vi "Choreo_Trajectory_SampleInternal.vi"(9 "TimeStamp":dbl, 11 "ChoreoTrajectory":T2) -> (3 "ChoreoTrajectoryState":T1)   [LabVIEW 2019, in "ChoreoLib.lvlib"]
doc: "This is an internal routine. It should NOT be called by the end user. Return an interpolated sample of the trajectory at the given timestamp.\n\nInputs: \n - ChoreoTrajectory - cluster - The trajectory to sample.\n - timestamp - double - The timestamp of this sample relative to the beginning of the trajectory.\n\nOutputs:\n - ChoreoTrajectoryState - cluster - The ChoreoTrajectoryState at the given time."
uses:
  ChoreoLib.lvlib
  TypeDef/ChoreoTrajectory.ctl
  TypeDef/ChoreoTrajectoryState.ctl
  Choreo_TrajectoryState_New.vi
  Choreo_TrajectoryState_GetAll.vi
  <vilib>/Rock Robotics/WPI/ThirdParty/JAS_Junk/TrajLib/Pose2d_Interpolate.vi
  Choreo_TrajectoryState_GetPose.vi
  <vilib>/Rock Robotics/WPI/ThirdParty/JAS_Junk/TrajLib/MathUtil_Interpolate.vi
  <vilib>/Rock Robotics/WPI/ThirdParty/JAS_Junk/TrajLib/Pose2d_getXYAngle.vi
  <vilib>/Rock Robotics/WPI/ThirdParty/JAS_Junk/TrajLib/Twist2d_GetAll.vi
  <vilib>/Rock Robotics/WPI/ThirdParty/JAS_Junk/TrajLib/Twist2d_Create.vi
  <vilib>/Rock Robotics/WPI/ThirdParty/JAS_Junk/TrajLib/Pose2d_New.vi
  <vilib>/Rock Robotics/WPI/ThirdParty/JAS_Junk/TrajLib/MathUtil_Clamp.vi
  <vilib>/Rock Robotics/WPI/ThirdParty/JAS_Junk/TrajLib/Rotation2d_CreateAngle.vi
  <vilib>/Rock Robotics/WPI/ThirdParty/JAS_Junk/TrajLib/Translation2d_Create.vi
  <vilib>/Rock Robotics/WPI/ThirdParty/JAS_Junk/TrajLib/Pose2d_Log.vi
  <vilib>/Rock Robotics/WPI/ThirdParty/JAS_Junk/TrajLib/Pose2d_Exp.vi
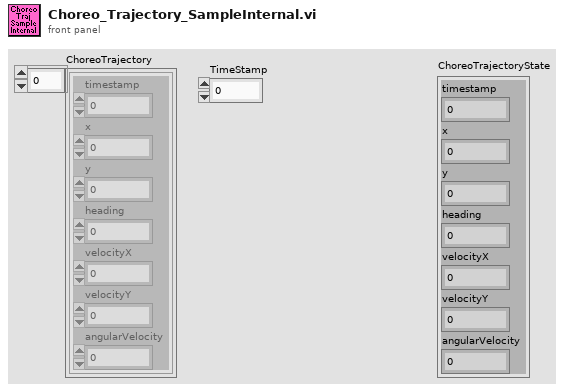
[diagram p1: front panel]
types:
  T1 = typedef "ChoreoLib.lvlib/ChoreoTrajectoryState.ctl" = cluster{"timestamp":dbl, "x":dbl, "y":dbl, "heading":dbl, "velocityX":dbl, "velocityY":dbl, "angularVelocity":dbl}
  T2 = typedef "ChoreoLib.lvlib/ChoreoTrajectory.ctl" = T1[]
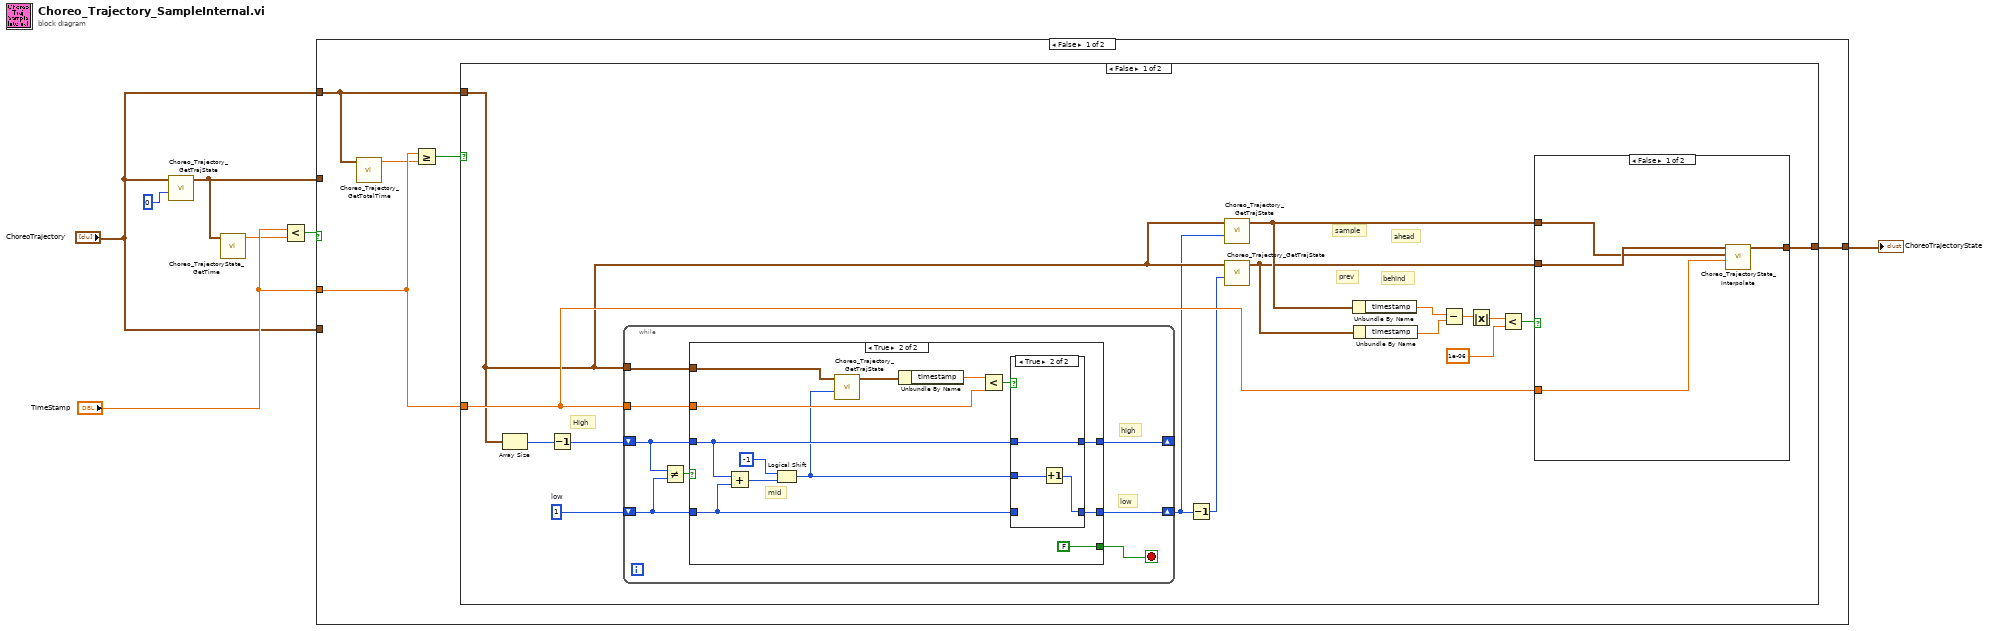
[diagram p0: block diagram]
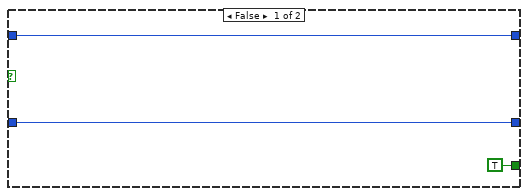
[diagram p3: hidden frame]
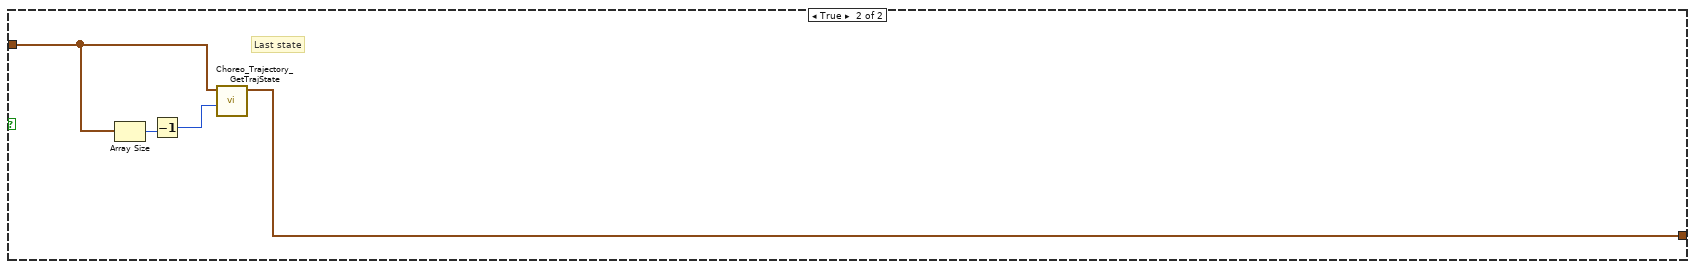
[diagram p5: hidden frame]
diagram:
  n1 = call "Choreo_Trajectory_GetTrajState.vi"("index"=0, "ChoreoTrajectory"="ChoreoTrajectory") -> ("ChoreoTrajectoryState"=w2:T1)  [unwired: 9 in]
  n2 = call "Choreo_TrajectoryState_GetTime.vi"("ChoreoTrajectoryState"=w2) -> ("timestamp"=w1:dbl)  [unwired: 10 in]
  n3 = Less?(x="TimeStamp", y=w1) -> (x < y?=w7:bool)
  n4 = case shown="False" w7 {
    tunnel: w2 -> [_ w67]
    tunnel: [w11 w67] -> w6
    tunnel: "ChoreoTrajectory" -> [w9 _]
    tunnel: "TimeStamp" -> [w10 _]
    tunnel: "ChoreoTrajectory" -> [_ _]
    frame False {
      n5 = call "Choreo_Trajectory_GetTotalTime.vi"("ChoreoTrajectory"=w9) -> ("TotalTime"=w8:dbl)  [unwired: 10 in]
      n6 = Greater Or Equal?(x=w10, y=w8) -> (x >= y?=w12:bool)
      n7 = case shown="False" w12 {
        tunnel: [w21 w63] -> w11
        tunnel: w9 -> [w17 w64]
        tunnel: w10 -> [w19 _]
        frame False {
          w26 = 1  # low
          # "ahead"
          # "behind"
          # "prev"
          # "sample"
          # "High"
          n8 = Array Size(array=w17) -> (size(s)=w28:i32)
          n9 = Decrement(x=w28) -> (x-1=w27:i32)
          n10 = while {
            shift-right: [w39] -> w16
            shift-left: w26 -> [w35]
            shift-right: [w40] -> _
            shift-left: w27 -> [w36]
            tunnel: w17 -> [w38]
            tunnel: w19 -> [w41]
            stop <- w34 stop-if-true
            # "high"
            # "low"
            n11 = Not Equal?(x=w36, y=w35) -> (x != y?=w37:bool)
            n12 = case shown="True" w37 {
              tunnel: w41 -> [_ w54]
              tunnel: w36 -> [w44 w52]
              tunnel: w35 -> [w43 w51]
              tunnel: [w44 w50] -> w40
              tunnel: [w43 w49] -> w39
              tunnel: w38 -> [_ w46]
              tunnel: [TRUE FALSE] -> w34
              frame False {
              }
              frame True {
                # "mid"
                n13 = Add(x=w52, y=w51) -> (x+y=w57:i32)
                n14 = Logical Shift(y=i16 -1, x=w57) -> (x << y=w47:i32)
                n15 = call "Choreo_Trajectory_GetTrajState.vi"("index"=w47, "ChoreoTrajectory"=w46) -> ("ChoreoTrajectoryState"=w45:T1)  [unwired: 9 in]
                n16 = Unbundle By Name(w45) -> ("timestamp"=w55:dbl)
                n17 = Less?(x=w55, y=w54) -> (x < y?=w53:bool)
                n18 = case shown="True" w53 {
                  tunnel: w52 -> [_ w62]
                  tunnel: [w58 w62] -> w50
                  tunnel: w47 -> [w58 w61]
                  tunnel: w51 -> [w59 _]
                  tunnel: [w59 w60] -> w49
                  frame False {
                  }
                  frame True {
                    n19 = Increment(x=w61) -> (x+1=w60:i32)
                  }
                }
              }
            }
          }
          n20 = Decrement(x=w16) -> (x-1=w15:i32)
          n21 = call "Choreo_Trajectory_GetTrajState.vi"("index"=w16, "ChoreoTrajectory"=w17) -> ("ChoreoTrajectoryState"=w14:T1)  [unwired: 9 in]
          n22 = call "Choreo_Trajectory_GetTrajState.vi"("index"=w15, "ChoreoTrajectory"=w17) -> ("ChoreoTrajectoryState"=w13:T1)  [unwired: 9 in]
          n23 = Unbundle By Name(w14) -> ("timestamp"=w18:dbl)
          n24 = Unbundle By Name(w13) -> ("timestamp"=w20:dbl)
          n25 = Subtract(x=w18, y=w20) -> (x-y=w25:dbl)
          n26 = Absolute Value(x=w25) -> (abs(x)=w24:dbl)
          n27 = Less?(x=w24, y=1e-06) -> (x < y?=w22:bool)
          n28 = case shown="False" w22 {
            tunnel: w14 -> [w30 w33]
            tunnel: [w29 w33] -> w21
            tunnel: w13 -> [w31 _]
            tunnel: w19 -> [w32 _]
            frame False {
              n29 = call "Choreo_TrajectoryState_Interpolate.vi"("T"=w32, "EndValue TrajectoryState"=w30, "ChoreoTrajectoryState"=w31) -> ("Interpolated ChoreoTrajectoryState"=w29:T1)  [unwired: 8 in]
            }
            frame True {
            }
          }
        }
        frame True {
          # "Last state"
          n30 = Array Size(array=w64) -> (size(s)=w66:i32)
          n31 = Decrement(x=w66) -> (x-1=w65:i32)
          n32 = call "Choreo_Trajectory_GetTrajState.vi"("index"=w65, "ChoreoTrajectory"=w64) -> ("ChoreoTrajectoryState"=w63:T1)  [unwired: 9 in]
        }
      }
    }
    frame True {
      # "First State"
    }
  }
  "ChoreoTrajectoryState" <- w6
